vi "pid-toolkit-online-autotuning.vi"() -> ()   [LabVIEW 2018, in "pid-toolkit.lvlib"]
uses:
  pid-toolkit.lvlib
  <vilib>/addons/control/pid/autopid.llb/PID autotuning parameters.ctl
  <vilib>/Platform/TimedLoop/XDataNode/timing_clust.ctl
  <vilib>/Platform/TimedLoop/XDataNode/nitl_modes.ctl
  <vilib>/Platform/TimedLoop/XDataNode/wakeup.ctl
  <vilib>/addons/control/pid/autopid.llb/PID Online Autotuning (Step Open Loop).vi
  <vilib>/addons/control/pid/autopid.llb/PID Online Autotuning (Step Closed Loop).vi
  <vilib>/addons/control/pid/autopid.llb/PID Online Autotuning (Relay Feedback).vi
  <vilib>/addons/control/pid/autopid.llb/PID Online Autotuning (PID on the loop).vi
  <vilib>/platform/TimedLoop/XDataNode/XDataNode.xnode
  <vilib>/Platform/TimedLoop/XDataNode/XDNodeRunTimeDep.lvlib
  <vilib>/addons/control/pid/NI_PID_autopid.lvlib
panel:
  in  "Clear Error":bool
  out "tuning completed?":bool
  out "Tuned PID Gains":T1={"proportional gain (Kc)"=1.0, "integral time (Ti, min)"=0.01, "derivative time (Td, min)"=0.0} {"derivative time (Td, min)" format="%.3f"; "integral time (Ti, min)" format="%.3f"; "proportional gain (Kc)" format="%.3f"}
  out "setpoint out":dbl(slide)=30.8641975308642 scale=0.0..100.0 scale format="%.1f"
  out "Process Variable Output":dbl(slide)=19.583333333333336 scale=0.0..100.0 scale format="%.1f"
  out "PID gains out":T1={"proportional gain (Kc)"=1.0, "integral time (Ti, min)"=0.01, "derivative time (Td, min)"=0.0} {"derivative time (Td, min)" format="%.3f"; "integral time (Ti, min)" format="%.3f"; "proportional gain (Kc)" format="%.3f"}
  in  "Reinitialize":bool
  in  "PID Gains Input":T1={"proportional gain (Kc)"=1.0, "integral time (Ti, min)"=0.01, "derivative time (Td, min)"=0.0} {"derivative time (Td, min)" format="%.3f"; "integral time (Ti, min)" format="%.3f"; "proportional gain (Kc)" format="%.3f"}
  in  "Autotuning Parameters":T2={"type of controller"=0, "relay cycles"=3, "relay amplitude"=1.0, "control specifications"=2, "PV noise level"=0.1} {"PV noise level" format="%.2f"; "control specifications" items=["normal", "fast", "slow"]; "relay amplitude" format="%.2f"; "type of controller" items=["P", "PI", "PID"]}
  in  "Setpoint":dbl(slide) scale=0.0..300.0
  out "Single Update (Multiple Plots, stacked)":cluster{"Temperature":sgl, "Setpoint":sgl, sgl}(graph)
  out "Output":u16
  out "High":bool
  out "Low":bool
  in  "Manual":u8(slide) scale=0.0..255.0
  in  "Method":T3(ring)
  out "Modbus error":errorcluster
  in  "Off Hook":bool
  in  "Update Rate":dbl caption="Rate"
  out "Failure":bool
  out "Updating":bool
  in  "Update Now":bool
  in  "Maximum":sgl
  in  "Minimum":sgl
  out "Thermometer":sgl(slide) scale=0.0..260.0
  in  "Force exit out of loop":bool
  out "Interval":i64
  out "Duration":i64
  out "Cycle":i32
  in  "Frequency":dbl(slide) scale=0.1..10.0
  # "Loop"
  # "Modbus"
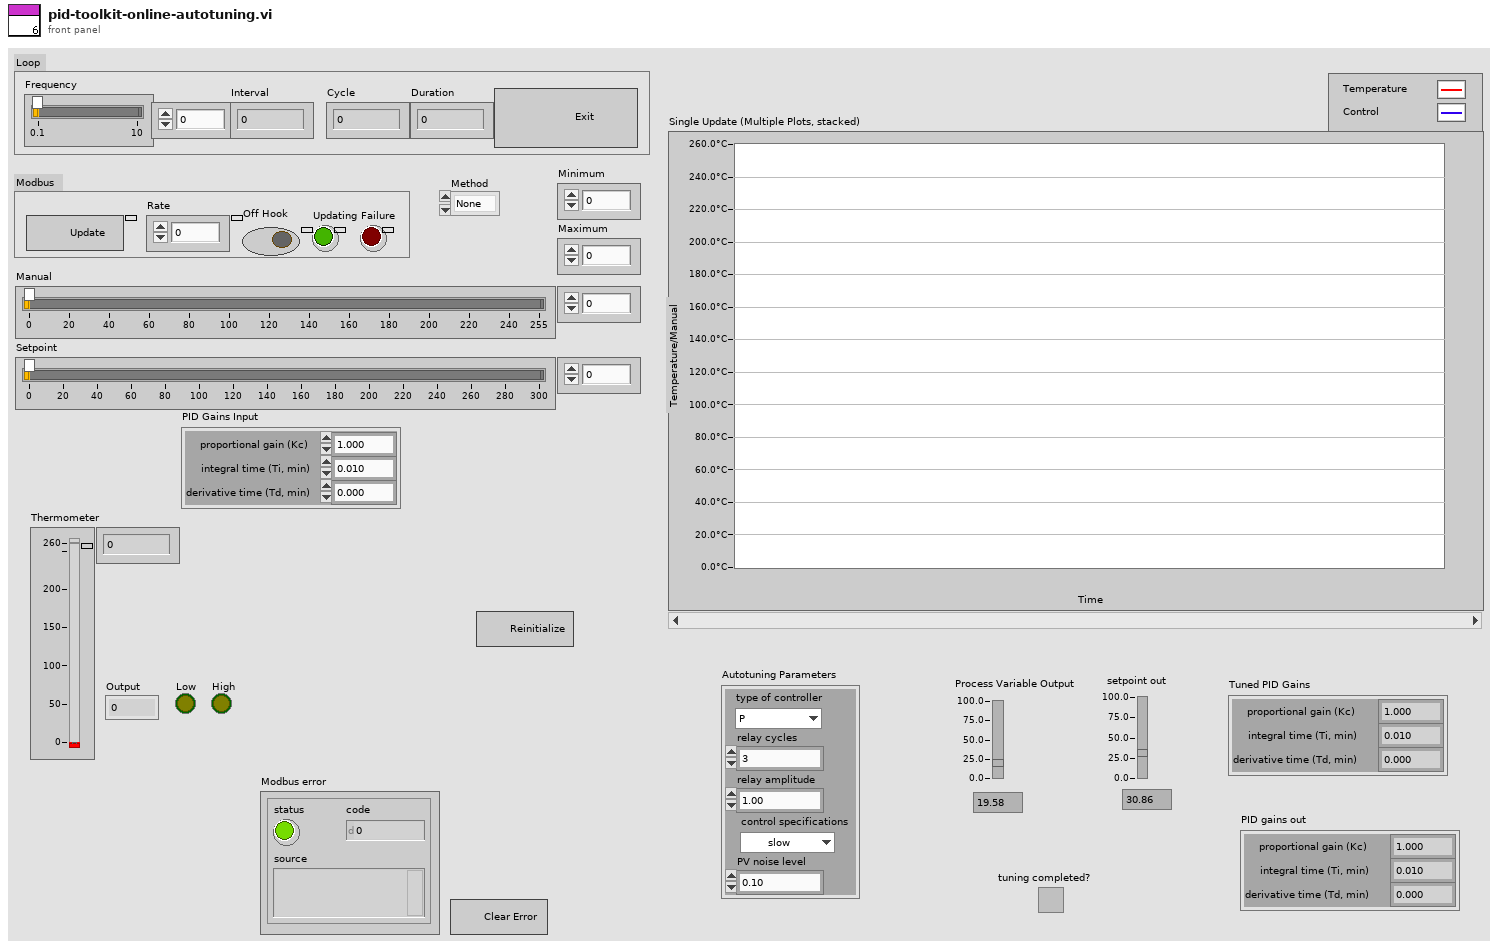
[diagram p1: front panel]
types:
  T1 = cluster{"proportional gain (Kc)":dbl, "integral time (Ti, min)":dbl, "derivative time (Td, min)":dbl}
  T2 = typedef "PID autotuning parameters.ctl" = cluster{"type of controller":u16, "relay cycles":i32, "relay amplitude":dbl, "control specifications":u16, "PV noise level":dbl}
  T3 = enum16{"None", "Step Open Loop", "Step Closed Loop", "Relay Feedback", "PID Relay"}
  T4 = typedef "XDNodeRunTimeDep.lvlib/timing_clust.ctl" = cluster{"Expected End [f-1]":u64, "Actual End [f-1]":u64, "Finished Late? [f-1]":bool, "Expected End [i-1]":u64, "Actual End [i-1]":u64, "Finished Late? [i-1]":bool, "Expected Start [i]":u64, "Actual Start [i]":u64, "Expected Start [f]":u64, "Actual Start [f]":u64, "Source Name":string, "Structure Name":string, "Period":i64, "Deadline":i64, "Offset":i64, "Start":i64, "Priority":i32, "Timeout":i32, "Mode":T5, "Wakeup Reason":T6, "Error":errorcluster, "Source Type":string, "Secondary Source Type":string, "Global End Time":u64, "Global Start Time":u64, "Frame Duration":u64, "Iteration Duration":u64, "Assigned CPU":i32, "I/O Scan Engine Mode":u32}
  T5 = typedef "XDNodeRunTimeDep.lvlib/nitl_modes.ctl" = enum32{"No Change", "Process missed periods, maintain original phase", "Discard missed periods, maintain original phase", "Process missed periods, ignore original phase", "Discard missed periods, ignore original phase"}
  T6 = typedef "XDNodeRunTimeDep.lvlib/wakeup.ctl" = enum32{"Normal", "Aborted", "Asynchronous wakeup", "Timing source error", "Timed loop error", "Timeout"}
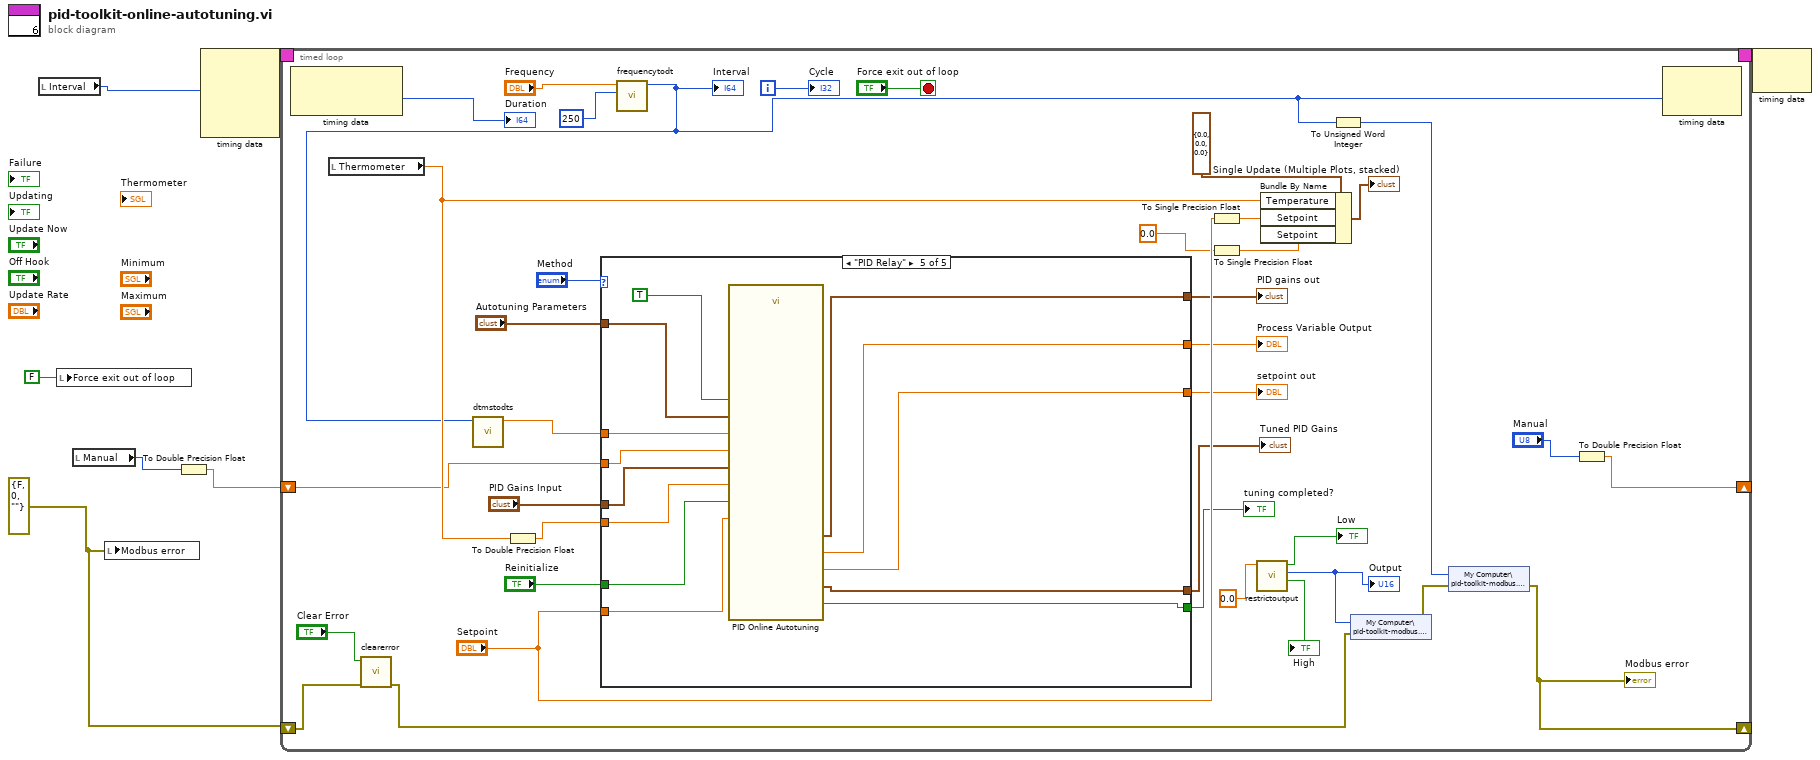
[diagram p0: block diagram]
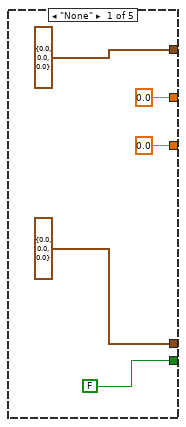
[diagram p2: hidden frame]
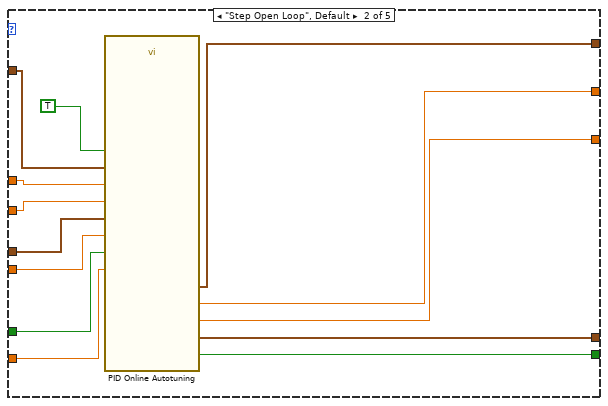
[diagram p3: hidden frame]
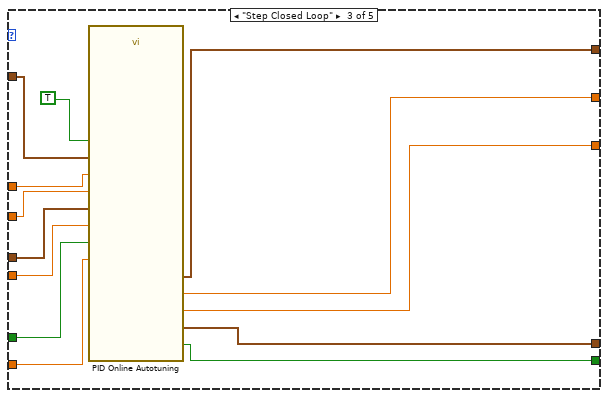
[diagram p4: hidden frame]
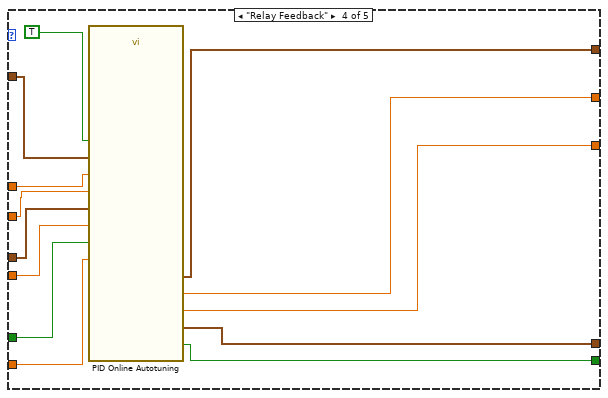
[diagram p5: hidden frame]
diagram:
  w3 = errorcluster {"status"=FALSE, "code"=0, "source"=""} ("Modbus error")
  n1 = local read "Interval"() -> (w4:i64)
  n2 = local write "Force exit out of loop"(FALSE ("Force exit out of loop")) -> ()
  n3 = local read "Manual"() -> (w1:u8)
  n4 = local write "Modbus error"(w3) -> ()
  n5 = To Double Precision Float(number=w1) -> (double precision float=w2:dbl)
  n6 = node-c288(w4) -> (w7:T4)  [unwired: 3 in]
  n7 = timed-loop {
    timing: w7 -> [_]
    timing-out: [_] -> w6
    shift-right: [w20] -> _
    shift-left: w3 -> [w19]
    shift-right: [w9] -> _
    shift-left: w2 -> [w10]
    i -> [w40]
    stop <- "Force exit out of loop" stop-if-true
    n8 = node-c288() -> (→"Duration":i64)  [unwired: 1 in, 1 out]
    n9 = local read "Thermometer"() -> (w33:sgl)
    n10 = call "clearerror.vi"("error in (no error)"=w19, "Clear Error"="Clear Error") -> ("error out"=w18:errorcluster)  [unwired: 9 in]
    n11 = To Double Precision Float(number=w33) -> (double precision float=w21:dbl)
    n12 = call "frequencytodt.vi"("Default in"=i64 250, "Frequency"="Frequency") -> ("Default out"=w30:i64)  [unwired: 9 in]
    "Interval" <- w30
    n13 = call "dtmstodts.vi"("Default in"=w30) -> ("Numeric"=w39:dbl)  [unwired: 10 in]
    n14 = case shown="\"PID Relay\"" "Method" {
      tunnel: w39 -> [_ w60 w73 w86 w99]
      tunnel: "Autotuning Parameters" -> [_ w61 w74 w87 w100]
      tunnel: "PID Gains Input" -> [_ w59 w72 w85 w97]
      tunnel: "Setpoint" -> [_ w58 w69 w82 w94]
      tunnel: "Reinitialize" -> [_ w57 w70 w83 w95]
      tunnel: w21 -> [_ w56 w71 w84 w96]
      tunnel: [T1 {"proportional gain (Kc)"=0.0, "integral time (Ti, min)"=0.0, "derivative time (Td, min)"=0.0} ("PID gains out") w55 w68 w81 w93] -> w16
      tunnel: [0.0 ("process variable out") w54 w67 w80 w92] -> w15
      tunnel: [0.0 ("setpoint out") w53 w66 w79 w91] -> w14
      tunnel: [T1 {"proportional gain (Kc)"=0.0, "integral time (Ti, min)"=0.0, "derivative time (Td, min)"=0.0} ("tuned PID gains") w52 w65 w78 w90] -> w13
      tunnel: [FALSE ("tuning completed?") w51 w64 w77 w89] -> w12
      tunnel: w10 -> [_ w50 w63 w76 w98]
      frame "None" {
      }
      frame "Step Open Loop", Default {
        n15 = call-poly <vilib>:"PID Online Autotuning.vi"("setpoint"=w58, "manipulated variable"=w50, "autotuning parameters"=w61, "process variable"=w56, "PID gains in"=w59, "dt (s)"=w60, "reinitialize? (F)"=w57, "autotune? (F)"=TRUE) -> ("setpoint out"=w53:dbl, "process variable out"=w54:dbl, "tuning completed?"=w51:bool, "PID gains out"=w55:T1, "tuned PID gains"=w52:T1)  [unwired: 3 in]
      }
      frame "Step Closed Loop" {
        n16 = call-poly <vilib>:"PID Online Autotuning.vi"("setpoint"=w69, "manipulated variable"=w63, "autotuning parameters"=w74, "process variable"=w71, "PID gains in"=w72, "dt (s)"=w73, "reinitialize? (F)"=w70, "autotune? (F)"=TRUE) -> ("setpoint out"=w66:dbl, "process variable out"=w67:dbl, "tuning completed?"=w64:bool, "PID gains out"=w68:T1, "tuned PID gains"=w65:T1)  [unwired: 3 in]
      }
      frame "Relay Feedback" {
        n17 = call-poly <vilib>:"PID Online Autotuning.vi"("setpoint"=w82, "manipulated variable"=w76, "autotuning parameters"=w87, "process variable"=w84, "PID gains in"=w85, "dt (s)"=w86, "reinitialize? (F)"=w83, "autotune? (F)"=TRUE) -> ("setpoint out"=w79:dbl, "process variable out"=w80:dbl, "tuning completed?"=w77:bool, "PID gains out"=w81:T1, "tuned PID gains"=w78:T1)  [unwired: 3 in]
      }
      frame "PID Relay" {
        n18 = call-poly <vilib>:"PID Online Autotuning.vi"("setpoint"=w94, "manipulated variable"=w98, "autotuning parameters"=w100, "process variable"=w96, "PID gains in"=w97, "dt (s)"=w99, "reinitialize? (F)"=w95, "autotune? (F)"=TRUE) -> ("setpoint out"=w91:dbl, "process variable out"=w92:dbl, "tuning completed?"=w89:bool, "PID gains out"=w93:T1, "tuned PID gains"=w90:T1)  [unwired: 3 in]
      }
    }
    "PID gains out" <- w16
    "Process Variable Output" <- w15
    "setpoint out" <- w14
    "Tuned PID Gains" <- w13
    "tuning completed?" <- w12
    n19 = To Single Precision Float(number="Setpoint") -> (single precision float=w28:sgl)
    n20 = To Single Precision Float(number=sgl 0.0) -> (single precision float=w27:sgl)
    n21 = call "restrictoutput.vi"("Input"=0.0) -> ("Hig"=→"High":bool, "Output"=w36:u16, "Low"=→"Low":bool)  [unwired: 8 in]
    "Output" <- w36
    n22 = Bundle By Name(cluster=cluster{"Temperature":sgl, "Setpoint":sgl, sgl} {"Temperature"=0.0, "Setpoint"=0.0, 0.0} ("Single Update (Multiple Plots, stacked)"), "Temperature"=w33, "Setpoint"=w28, "Setpoint"=w27) -> (→"Single Update (Multiple Plots, stacked)":cluster{"Temperature":sgl, "Setpoint":sgl, sgl})
    n23 = To Unsigned Word Integer(number=w30) -> (unsigned 16bit integer=w31:u16)
    n24 = shared-variable "My Computer\\pid-toolkit-modbus.lvlib\\400002"(w36, error in=w18) -> (error out=w32:errorcluster)
    n25 = shared-variable "My Computer\\pid-toolkit-modbus.lvlib\\400001"(w31, error in=w32) -> (error out=w20:errorcluster)
    "Modbus error" <- w20
    n26 = To Double Precision Float(number="Manual") -> (double precision float=w9:dbl)
    n27 = node-c288(w30) -> ()  [unwired: 1 in, 1 out]
    "Cycle" <- w40
  }
  n28 = node-c288(w6) -> ()  [unwired: 1 out]
